vi "Ohaus AV Series Single Measurement.vi"(1 "Units (0: Gram)":u16(ring) items=["Gram (g)"=0, "Kilogram (kg)"=1, "Penny weight (dwt)"=2, "Carat (ct)"=3, "Ounce (oz)"=4, "Ounce Troy (oz t)"=5, "Grain (GN)"=6, "Hong Kong Tael (HKt)"=7, "Singapore Tael (SGt)"=8, "Tiwan Tael (TWt)"=9, "Momme (m)"=10, "Pound (lb)"=11, "Newton (N)"=13, "Tical (ti)"=14, "Tula"=15, "Mesghal (Meshg)"=16, "Baht"=17, "Custom"=19], 2 "VISA resource name":refnum<visa-resource-name>="COM7", 3 "Serial Configuration":T1={"Baud Rate (2400)"=9600, "Flow Control (1: XON/XOFF)"=2, "Parity (0: None)"=0, "Data Bits (7)"=8} {"Data Bits (7)" items=["7"=7, "8"=8]; "Parity (0: None)" items=["None", "Odd", "Even"]; "Flow Control (1: XON/XOFF)" items=["None", "XON/XOFF", "RTS/CTS"]; "Baud Rate (2400)" items=["600"=600, "1200"=1200, "2400"=2400, "4800"=4800, "9600"=9600, "19200"=19200]}) -> (0 "Weight Value":dbl format="%#.3g")   [LabVIEW 2015]
doc: "This VI will take a single measurement in the units selected.\n\n<B>Before running this VI some initial instrument setup is required:</B>\nOnly Gross, Net, Tare; Reference; and GLP need to be changed from their default values to OFF\n\nGoto the menu screen on the balance\n Then the PRINT-1 menu\n \n Output\n When Stable: OFF (default) \n GLP Tare: OFF (default)\n Auto Print: OFF (default)\n Content\n Number Only: OFF (default)\n Header: OFF (default)\n<B> Gross, Net, and Tare: OFF</B>\n<B> Reference: OFF</B>\n Result: ON (default)\n<B> GLP: OFF</B>\n Layout\n Line Format: MULTI (default)\n Line Feed: OFF (default)\n Form Feed: OFF (default)"
uses:
  Ohaus AV Series.lvlib
panel:
  out "Stable?":bool
  out "NET":bool
  out "Units":string
  # "(c) 2004-2009 National Instruments.  All Rights Reserved."
  # "Before running this VI some initial setup is required\n(See VI documentation for more information)"
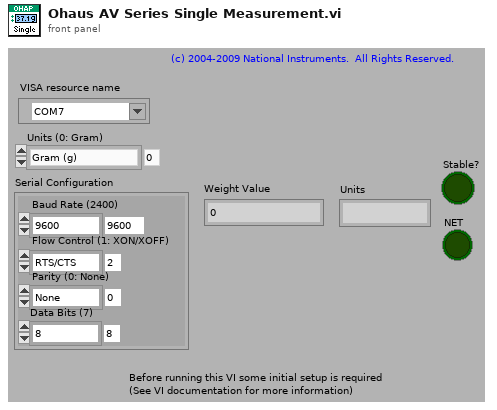
[diagram p1: front panel]
types:
  T1 = cluster{"Baud Rate (2400)":u32, "Flow Control (1: XON/XOFF)":u16, "Parity (0: None)":u16, "Data Bits (7)":u16}
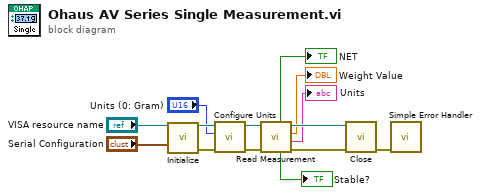
[diagram p0: block diagram]
diagram:
  n1 = call "Initialize.vi"("VISA resource name"="VISA resource name", "Serial Configuration"="Serial Configuration") -> ("VISA resource name out"=w13:refnum<visa-resource-name>, "error out"=w14:errorcluster)  [unwired: 12 in]
  n2 = call "Configure Units.vi"("error in (no error)"=w14, "Units (0: Gram)"="Units (0: Gram)", "VISA resource name"=w13) -> ("error out"=w12:errorcluster, "VISA resource name out"=w11:refnum<visa-resource-name>)  [unwired: 7 in]
  n3 = call "Read Measurement.vi"("error in (no error)"=w12, "VISA resource name"=w11) -> ("error out"=w10:errorcluster, "Units"=→"Units":string, "Weight Value"=→"Weight Value":dbl, "VISA resource name out"=w9:refnum<visa-resource-name>, "Stable?"=→"Stable?":bool, "NET"=→"NET":bool)  [unwired: 4 in]
  n4 = call "Close.vi"("error in (no error)"=w10, "VISA resource name"=w9) -> ("error out"=w4:errorcluster)  [unwired: 9 in]
  n5 = call <vilib>:"Simple Error Handler.vi"("error in (no error)"=w4) -> ()  [unwired: 4 in, 5 out]
